vi "Read Maximum Channel Duration.vi"(8 "error in (no error)":errorcluster, 11 "Waveforms (N Ch) in":refnum<class "Waveforms (N Ch).lvclass">) -> (0 "error out":errorcluster, 2 "maximum data duration (s)":dbl, 3 "Waveforms (N Ch) out":refnum<class "Waveforms (N Ch).lvclass">)   [LabVIEW 2017, in "Waveforms (N Ch).lvclass"]
uses:
  <vilib>/addons/_NISVFA/_Shared subVIs/Data Objects/Waveforms (DBL)/Waveforms (N Ch).lvclass
  C:/Program Files (x86)/National Instruments/LabVIEW 2017/vi.lib/addons/_NISVFA/_Shared subVIs/Data Objects/Data/Data.lvclass
  <vilib>/addons/_NISVFA/_Shared subVIs/Data Objects/Data/Data.lvclass/Data.ctl
  <vilib>/addons/_NISVFA/_Shared subVIs/Data Objects/Data/Data.lvclass
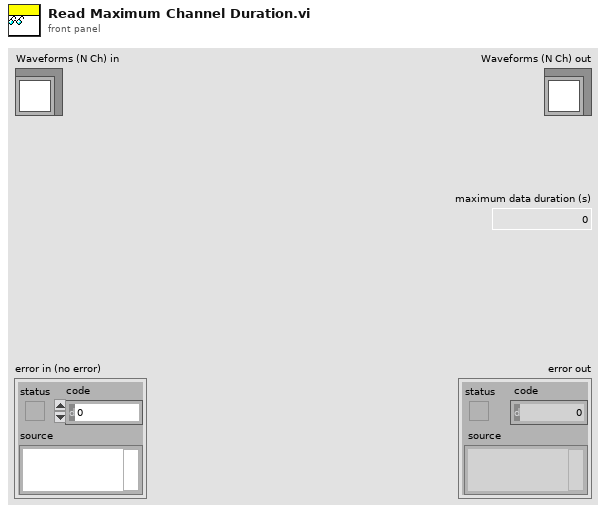
[diagram p1: front panel]
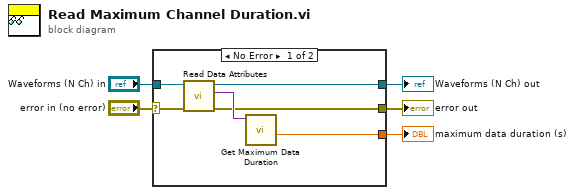
[diagram p0: block diagram]
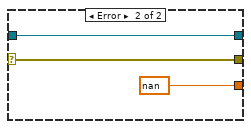
[diagram p2: hidden frame]
diagram:
  n1 = case shown="No Error" "error in (no error)" {
    selector: "error in (no error)" -> [w7 w13]
    tunnel: [w6 w13] -> w4
    tunnel: [w11 w14] -> w2
    tunnel: "Waveforms (N Ch) in" -> [w10 w14]
    tunnel: [w8 nan ("maximum data duration")] -> w1
    frame No Error {
      n2 = call <vilib>:"Read Data Attributes.vi"("error in (no error)"=w7, "Data in"=w10) -> ("error out"=w6:errorcluster, "data attributes"=w9:variant, "Data out"=w11:refnum<class "Waveforms (N Ch).lvclass">)  [unwired: 7 in]
      n3 = call <vilib>:"Get Maximum Data Duration.vi"("variant in"=w9) -> ("maximum data duration"=w8:dbl)  [unwired: 9 in, 1 out]
    }
    frame Error {
    }
  }
  "error out" <- w4
  "Waveforms (N Ch) out" <- w2
  "maximum data duration (s)" <- w1
